vi "Read Channel List.vi"(8 "error in":errorcluster, 11 "CoreOOB_Tx in":refnum<class "CIFCoreOOB_Tx.lvclass">) -> (0 "error out":errorcluster, 2 "Channel List":map{string, T1}(c390), 3 "CoreOOB_Tx out":refnum<class "CIFCoreOOB_Tx.lvclass">)   [LabVIEW 2021, in "CIFCoreOOB_Tx.lvclass"]
uses:
  CIFCoreOOB_Tx.lvclass
  D:/dev/CIF-LVCore/src/CIFUtilities/CIFOutOfBand/CIFOutOfBand.lvclass
  CIFUtilities/CIFChannelMng/typedef/Channel List for OOB.ctl
  CIFUtilities/CIFChannels/Typedef/Direction.ctl
  CIFUtilities/CIFOutOfBand/CIFOutOfBand.lvclass/CIFOutOfBand.ctl
  CIFUtilities/CIFOutOfBand/Accessors/Read Local OOB Data.vi
  CIFUtilities/CIFChannels/CIFChannels.lvclass
  CIFUtilities/CIFChannelMng/CIFChannelMng.lvclass
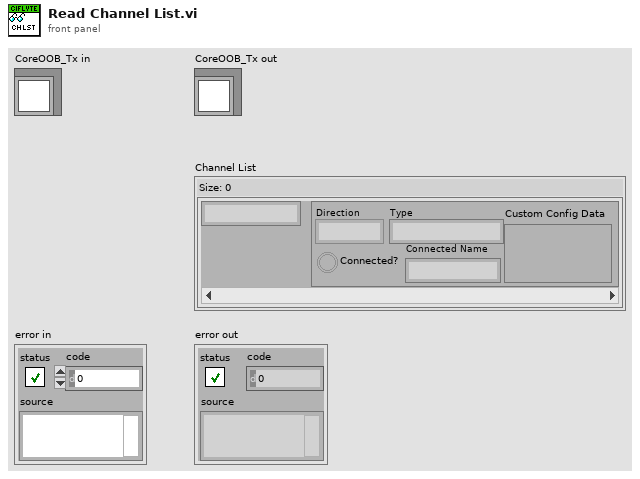
[diagram p1: front panel]
types:
  T1 = typedef "CIFChannelMng.lvclass/Channel List for OOB.ctl" = cluster{"Direction":T2, "Type":string, "Custom Config Data":variant, "Connected?":bool, "Connected Name":string}
  T2 = typedef "CIFChannels.lvclass/Direction.ctl" = enum16{"Publisher", "Subscriber"}
  T3 = typedef "CIFCoreOOB_Tx.lvclass/Template Payload.ctl" = cluster{"Status":T4, "Plugin Overrides":T13, "Channel List":map{string, T1}}
  T4 = typedef "CIFCoreCommon.lvlib/Plugin Status.ctl" = cluster{"State":T5, "Timing Statistics (us)":T6, "FIFO Statistics (us)":T8, "error":T9, "Monitor Doubles":T10, "Monitor U64":T11, "Monitor I64":T12, "Cleanup":T7, "Create":i32, "Destroy":i32}
  T5 = typedef "CIFCoreCommon.lvlib/Plugin State.ctl" = enum32{"Null", "Creating", "Listening", "Running", "CleaningUp", "Destroying"}
  T6 = typedef "CIFCoreCommon.lvlib/Timing Statistics.ctl" = cluster{"Period":T7, "Wake Error":T7, "Execute":T7, "Housekeep":T7, "Idle":T7}
  T7 = typedef "CIFCoreCommon.lvlib/Timing Stats Base.ctl" = cluster{"Max":i32, "Min":i32}
  T8 = typedef "CIFCoreCommon.lvlib/FIFO Statistics.ctl" = cluster{"From T0":T7, "From Previous Plugin":T7, "Output Error":T7}
  T9 = typedef "CIFCoreCommon.lvlib/Simple Error.ctl" = cluster{"status":bool, "code":i32}
  T10 = typedef "CIFCoreCommon.lvlib/Monitor Doubles.ctl" = cluster{"1":dbl, "2":dbl, "3":dbl, "4":dbl}
  T11 = typedef "CIFCoreCommon.lvlib/Monitor U64.ctl" = cluster{"1":u64, "2":u64, "3":u64, "4":u64}
  T12 = typedef "CIFCoreCommon.lvlib/Monitor I64.ctl" = cluster{"1":i64, "2":i64, "3":i64, "4":i64}
  T13 = typedef "CIFCoreCommon.lvlib/Plugin Overrides.ctl" = cluster{"Timing Overrides":T14}
  T14 = typedef "CIFCoreCommon.lvlib/Timing Overrides.ctl" = cluster{"Override Timing":bool, "Skip Sleep":bool, "Period (s)":dbl}
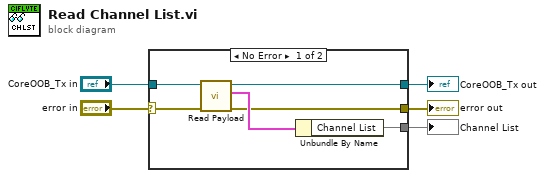
[diagram p0: block diagram]
diagram:
  n1 = case shown="No Error" "error in" {
    selector: "error in" -> [w7 w12]
    tunnel: [w6 w12] -> w4
    tunnel: [w10 w13] -> w2
    tunnel: "CoreOOB_Tx in" -> [w11 w13]
    tunnel: [w8 _] -> w1
    frame No Error {
      n2 = call "Read Payload.vi"("error in"=w7, "CoreOOB_Tx in"=w11) -> ("error out"=w6:errorcluster, "data"=w9:T3, "CoreOOB_Tx out"=w10:refnum<class "CIFCoreOOB_Tx.lvclass">)  [unwired: 7 in]
      n3 = Unbundle By Name(w9) -> ("Channel List"=w8:map{string, T1})
    }
    frame Error {
    }
  }
  "error out" <- w4
  "CoreOOB_Tx out" <- w2
  "Channel List" <- w1
